vi "Cycles.vi"() -> ()   [LabVIEW 2018]
uses:
  Spels.AutomationTools.RemoteFunctionalControlService.dll
panel:
  out "FPGA OE":bool
  in  "stop":bool
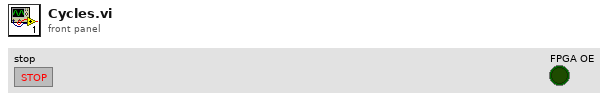
[diagram p1: front panel]
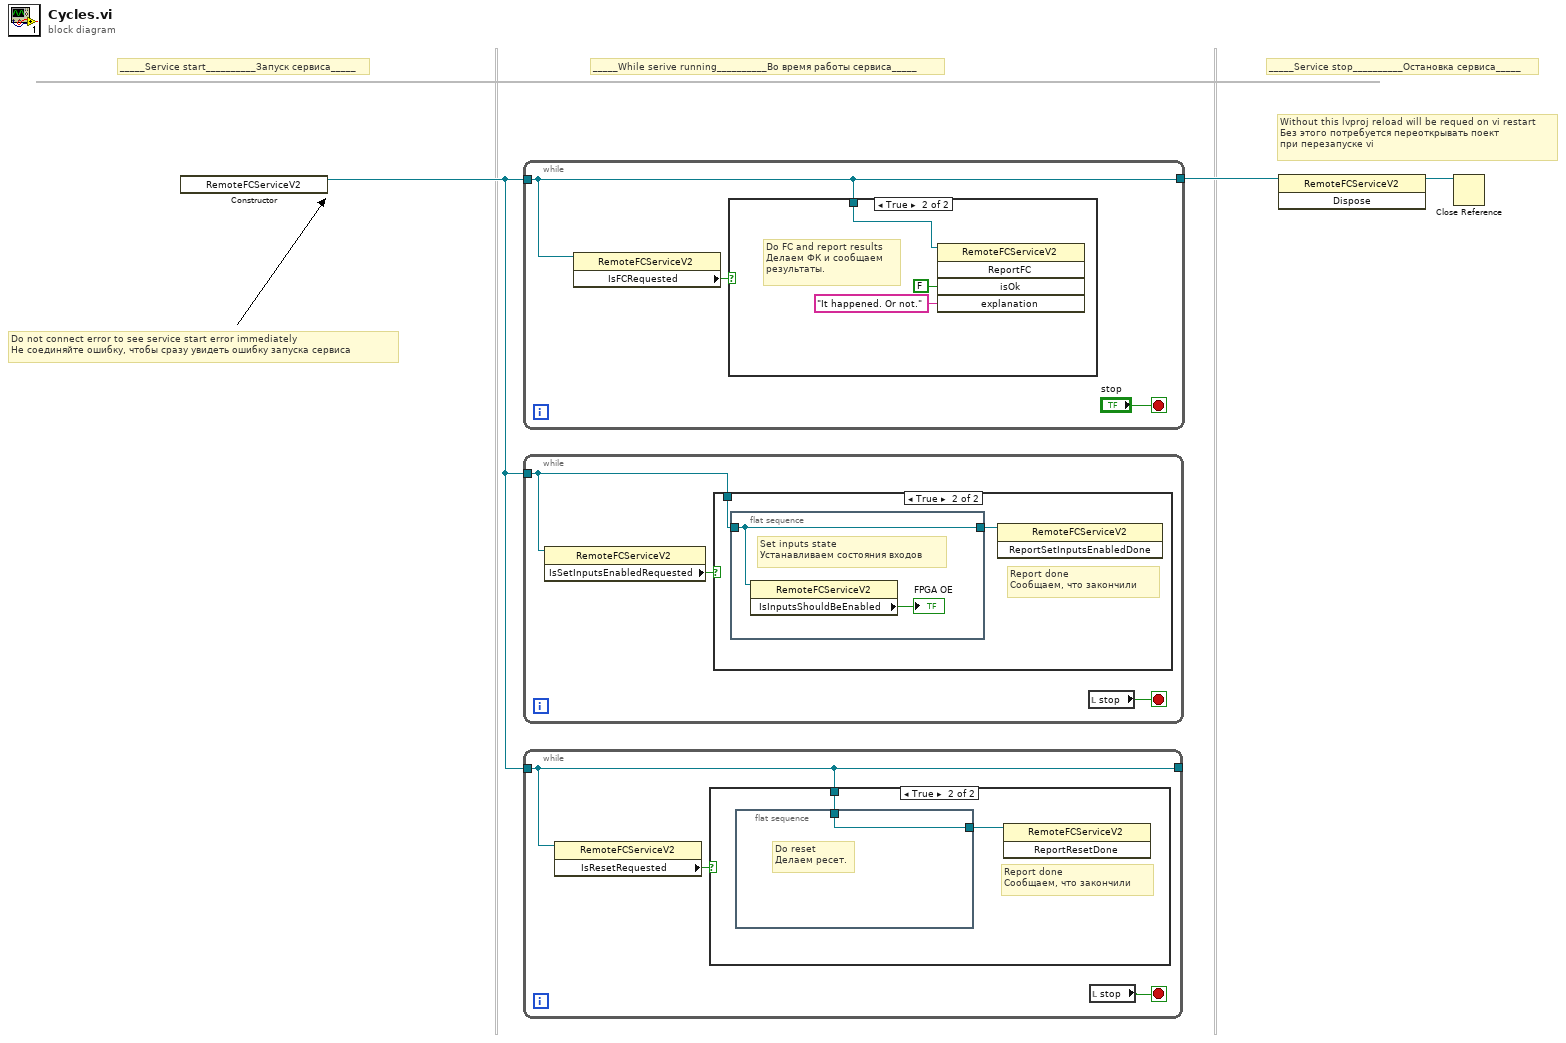
[diagram p0: block diagram]
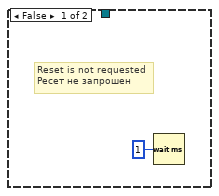
[diagram p2: hidden frame]
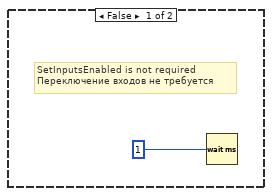
[diagram p3: hidden frame]
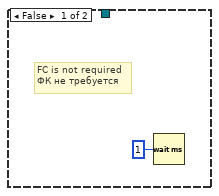
[diagram p4: hidden frame]
diagram:
  # "Do not connect error to see service start error immediately\nНе соединяйте ошибку, чтобы сразу увидеть ошибку запуска сервиса"
  # "Without this lvproj reload will be requed on vi restart\nБез этого потребуется переоткрывать поект \nпри перезапуске vi"
  # "_____Service stop__________Остановка сервиса_____"
  # "_____While serive running__________Во время работы сервиса_____"
  # "_____Service start__________Запуск сервиса_____"
  n1 = constructor class="RemoteFCServiceV2"() -> (reference out=w2:refnum<k24>)  [unwired: 3 in, 2 out]
  n2 = while {
    tunnel: [w5] -> w1
    tunnel: w2 -> [w5]
    stop <- "stop" stop-if-true
    n3 = property class="RemoteFCServiceV2"(reference=w5) -> ("IsFCRequested"=w4:bool)  [unwired: 1 in, 2 out]
    n4 = case shown="True" w4 {
      tunnel: w5 -> [_ w8]
      frame False {
        # "FC is not required\nФК не требуется"
        n5 = Wait (ms)(milliseconds to wait=u32 1) -> ()  [unwired: 1 out]
      }
      frame True {
        # "Do FC and report results\nДелаем ФК и сообщаем\nрезультаты."
        n6 = invoke class="RemoteFCServiceV2" method="ReportFC"(reference=w8, "isOk"=FALSE, "explanation"="It happened. Or not.") -> ()  [unwired: 2 in, 5 out]
      }
    }
  }
  n7 = while {
    tunnel: w2 -> [w13]
    stop <- w11 stop-if-true
    n8 = property class="RemoteFCServiceV2"(reference=w13) -> ("IsSetInputsEnabledRequested"=w12:bool)  [unwired: 1 in, 2 out]
    n9 = case shown="True" w12 {
      tunnel: w13 -> [_ w16]
      frame False {
        # "SetInputsEnabled is not required\nПереключение входов не требуется"
        n10 = Wait (ms)(milliseconds to wait=u32 1) -> ()  [unwired: 1 out]
      }
      frame True {
        # "Report done\nСообщаем, что закончили"
        n11 = flat-sequence {
          tunnel: w16 -> [w17]
          tunnel: [w17] -> w15
          frame #0 {
            # "Set inputs state\nУстанавливаем состояния входов"
            n12 = property class="RemoteFCServiceV2"(reference=w17) -> ("IsInputsShouldBeEnabled"=→"FPGA OE":bool)  [unwired: 1 in, 2 out]
          }
        }
        n13 = invoke class="RemoteFCServiceV2" method="ReportSetInputsEnabledDone"(reference=w15) -> ()  [unwired: 2 in, 3 out]
      }
    }
    n14 = local read "stop"() -> (w11:bool)
  }
  n15 = while {
    tunnel: [w21] -> _
    tunnel: w2 -> [w21]
    stop <- w19 stop-if-true
    n16 = property class="RemoteFCServiceV2"(reference=w21) -> ("IsResetRequested"=w20:bool)  [unwired: 1 in, 2 out]
    n17 = case shown="True" w20 {
      tunnel: w21 -> [_ w23]
      frame False {
        # "Reset is not requested\nРесет не запрошен"
        n18 = Wait (ms)(milliseconds to wait=u32 1) -> ()  [unwired: 1 out]
      }
      frame True {
        # "Report done\nСообщаем, что закончили"
        n19 = flat-sequence {
          tunnel: [w25] -> w24
          tunnel: w23 -> [w25]
          frame #0 {
            # "Do reset\nДелаем ресет."
          }
        }
        n20 = invoke class="RemoteFCServiceV2" method="ReportResetDone"(reference=w24) -> ()  [unwired: 2 in, 3 out]
      }
    }
    n21 = local read "stop"() -> (w19:bool)
  }
  n22 = invoke class="RemoteFCServiceV2" method="Dispose"(reference=w1) -> (reference out=w3:refnum<k24>)  [unwired: 2 in, 2 out]
  n23 = Close Reference(reference=w3) -> ()  [unwired: 1 in, 1 out]
